vi "Global - UI Loop Running.vi"() -> ()   [LabVIEW 2017]
panel:
  in  "UI Loop Running":bool
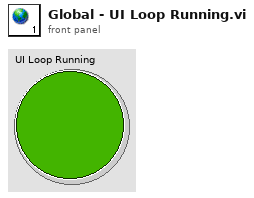
[diagram p1: front panel]
diagram:
